vi "Output File (Write).vi"(8 "error in (no error)":errorcluster, 10 "output_file":path, 11 "obj in":refnum<class "RequestBuilder.lvclass">) -> (0 "error out":errorcluster, 2 "success":bool, 3 "obj out":refnum<class "RequestBuilder.lvclass">)   [LabVIEW 2020, in "reqwest.lvlib" / "RequestBuilder.lvclass"]
uses:
  RequestBuilder.lvclass
  RequestBuilder.lvclass/RequestBuilder.ctl
  lv_reqwest_64.dll
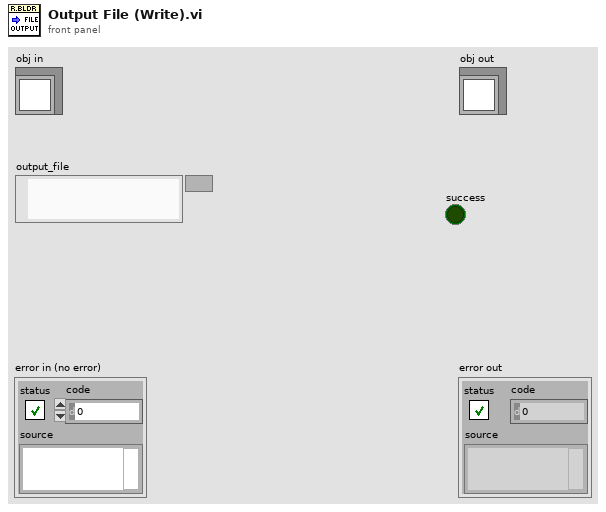
[diagram p1: front panel]
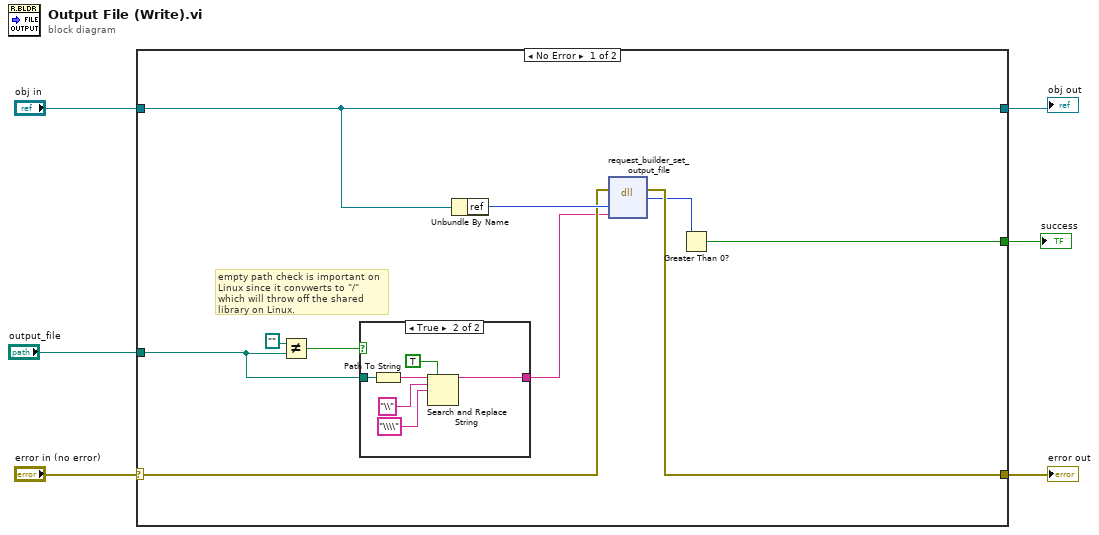
[diagram p0: block diagram]
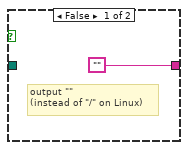
[diagram p2: hidden frame]
diagram:
  n1 = case shown="No Error" "error in (no error)" {
    selector: "error in (no error)" -> [w13 w24]
    tunnel: "obj in" -> [w14 w25]
    tunnel: [w16 w24] -> w3
    tunnel: [w14 w25] -> w4
    tunnel: "output_file" -> [w7 _]
    tunnel: [w11 _] -> w1
    frame No Error {
      # "empty path check is important on Linux since it convwerts to \"/\" which will throw off the shared library on Linux."
      n2 = Not Equal?(x=path "", y=w7) -> (x != y?=w10:bool)
      n3 = case shown="True" w10 {
        tunnel: w7 -> [_ w19]
        tunnel: ["" w18] -> w8
        frame False {
          # "output \"\"\n(instead of \"/\" on Linux)"
        }
        frame True {
          n4 = Path To String(path=w19) -> (string=w23:string)
          n5 = Search and Replace String(replace all?=TRUE ("replace all? (F)"), input string=w23, search string="\\", replace string="\\\\" ("replace string (\"\")")) -> (result string=w18:string)  [unwired: 4 in, 3 out]
        }
      }
      n6 = Unbundle By Name(w14) -> ("ref"=w15:u64)
      n7 = dll-call lib="C:/Projects/reqwest-rs-labview/lv_src/lv_reqwest_*.*" fn="request_builder_set_output_file"(error in=w13, "request_builder_ref"=w15, "output_file"=w8) -> (error out=w16:errorcluster, "success"=w12:u8)  [unwired: 4 in, 1 out]
      n8 = Greater Than 0?(x=w12) -> (x > 0?=w11:bool)
    }
    frame Error {
    }
  }
  "error out" <- w3
  "obj out" <- w4
  "success" <- w1
